vi "Read out parameter.vi"(5 "Board parameter? (F)":bool, 7 "All Channels (F)":bool, 8 "error in (no error)":errorcluster, 9 "Parameter name":string, 10 "Channel":u8, 11 "BoardHandle":T1) -> (0 "error out":errorcluster, 2 "Output values":string[](array[string]), 3 "BoardHandle out":T1)   [LabVIEW 2020, in "CAEN PSM.lvlib"]
doc: "This function allows reading a parameter indicated in the input (both of board and channel). The value will be returned as a string."
uses:
  CAEN PSM.lvlib
  BoardHandle.ctl
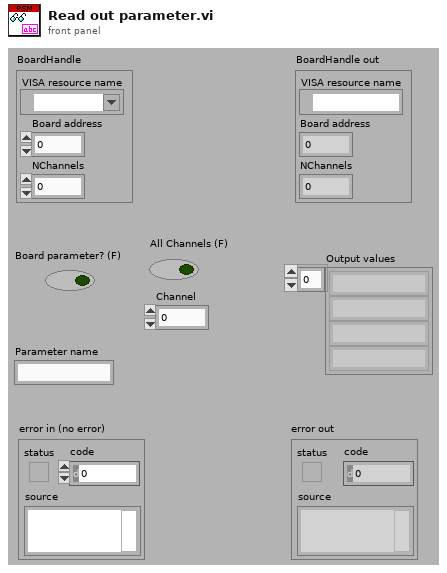
[diagram p1: front panel]
types:
  T1 = typedef "CAEN PSM.lvlib/BoardHandle.ctl" = cluster{"VISA resource name":refnum<visa-resource-name>, "Board address":i8, "NChannels":u8}
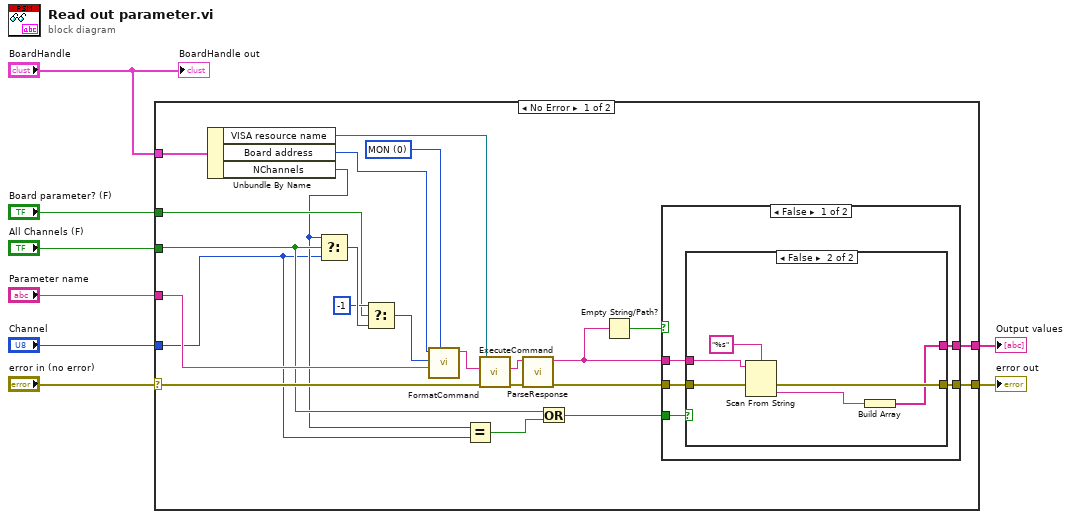
[diagram p0: block diagram]
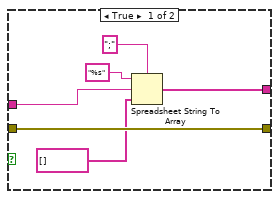
[diagram p2: hidden frame]
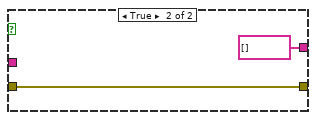
[diagram p3: hidden frame]
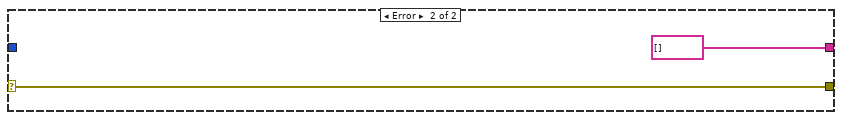
[diagram p4: hidden frame]
diagram:
  n1 = case shown="No Error" "error in (no error)" {
    selector: "error in (no error)" -> [w24 w52]
    tunnel: "All Channels (F)" -> [w14 _]
    tunnel: "Channel" -> [w11 _]
    tunnel: [w22 w52] -> w5
    tunnel: "BoardHandle" -> [w25 _]
    tunnel: [w21 string[] []] -> w3
    tunnel: "Board parameter? (F)" -> [w17 _]
    tunnel: "Parameter name" -> [w20 _]
    frame No Error {
      w30 = u8 0 items=["MON", "SET"] ("CMD")
      n2 = Unbundle By Name(w25) -> ("VISA resource name"=w29:refnum<visa-resource-name>, "Board address"=w31:i8, "NChannels"=w12:u8)
      n3 = Select(t=w12, s=w14, f=w11) -> (s? t:f=w19:u8)
      n4 = Select(t=i8 -1, s=w17, f=w19) -> (s? t:f=w16:u8)
      n5 = call "FormatCommand.vi"("CMD (MON)"=w30, "PAR"=w20, "CH"=w16, "BD (0)"=w31) -> ("cmd"=w28:string)  [unwired: 7 in]
      n6 = Equal?(x=w12, y=w11) -> (x = y?=w13:bool)
      n7 = call "ExecuteCommand.vi"("error in (no error)"=w24, "Command"=w28, "VISA resource name"=w29) -> ("error out"=w27:errorcluster, "Response"=w26:string)  [unwired: 6 in, 1 out]
      n8 = call "ParseResponse.vi"("error in (no error)"=w27, "Response"=w26) -> ("error out"=w23:errorcluster, "val"=w10:string)  [unwired: 6 in, 2 out]
      n9 = Or(x=w14, y=w13) -> (x .or. y?=w15:bool)
      n10 = Empty String/Path?(string/path=w10) -> (empty?=w9:bool)
      n11 = case shown="False" w9 {
        tunnel: w10 -> [w36 _]
        tunnel: w23 -> [w35 w50]
        tunnel: [w34 w50] -> w22
        tunnel: [w33 string[] []] -> w21
        tunnel: w15 -> [w32 _]
        frame False {
          n12 = case shown="False" w32 {
            tunnel: w36 -> [w39 w48]
            tunnel: w35 -> [w42 w46]
            tunnel: [w42 w45] -> w34
            tunnel: [w37 w44] -> w33
            frame True {
              n13 = Spreadsheet String To Array(delimiter (Tab)=";", format string="%s", spreadsheet string=w39, array type (2D Dbl)=string[] []) -> (array=w37:string[])
            }
            frame False {
              n14 = Scan From String(format string="%s", input string=w48, error in=w46) -> (error out=w45:errorcluster, output 1=w43:string)  [unwired: 2 in, 2 out]
              n15 = Build Array(w43) -> (w44:string[])
            }
          }
        }
        frame True {
        }
      }
    }
    frame Error {
    }
  }
  "error out" <- w5
  "Output values" <- w3
  "BoardHandle out" <- "BoardHandle"
